vi "GenBlink.vi"(5 "Color 2":u32(colorbox), 6 "Reset":bool, 7 "Color 1":u32(colorbox)=16711680, 10 "Period (ms)":i32=500, 11 "NumLeds":i32) -> (2 "Iterator":i32, 3 "Array":u32[](array[numeric]))   [LabVIEW 2018, in "ArduinoSerialBling.lvlib"]
uses:
  ArduinoSerialBling.lvlib
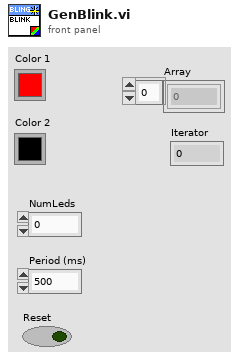
[diagram p1: front panel]
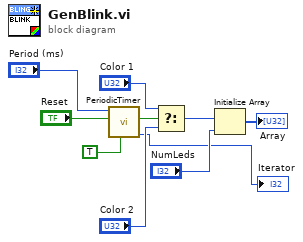
[diagram p0: block diagram]
diagram:
  n1 = call "PeriodicTimer.vi"("Initial"=TRUE, "Reset"="Reset", "Period (ms)"="Period (ms)") -> ("Iterator"=→"Iterator":i32, "Square Wave"=w7:bool)  [unwired: 6 in, 1 out]
  n2 = Select(t="Color 1", s=w7, f="Color 2") -> (s? t:f=w9:u32)
  n3 = Initialize Array(w9, "NumLeds") -> (→"Array":u32[])
